vi "General Commands.vi"(8 "error in":errorcluster, 9 "Current Limit":i32=1000, 10 "Action":T1, 11 "VISA in":refnum<visa-resource-name>) -> (0 "error out":errorcluster, 2 "result string":string, 3 "VISA out":refnum<visa-resource-name>)   [LabVIEW 2018]
uses:
  General_lecroy_command.ctl
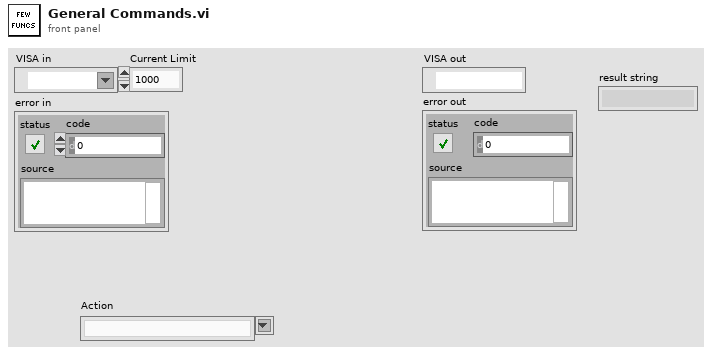
[diagram p1: front panel]
types:
  T1 = typedef "General_lecroy_command.ctl" = string
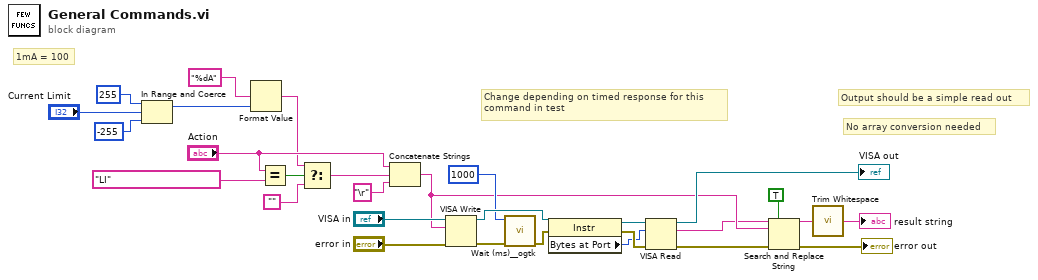
[diagram p0: block diagram]
diagram:
  # "1mA = 100"
  # "Change depending on timed response for this\ncommand in test"
  # "No array conversion needed"
  # "Output should be a simple read out"
  n1 = In Range and Coerce(upper limit=255, x="Current Limit", lower limit=-255 ("upper limit")) -> (coerced(x)=w3:i32)  [unwired: 1 out]
  n2 = Format Value(format string="%dA", value (0)=w3) -> (output string=w7:string)  [unwired: 1 in]
  n3 = Equal?(x="Action", y=T1 "LI") -> (x = y?=w10:bool)
  n4 = Select(t=w7, s=w10, f="") -> (s? t:f=w8:string)
  n5 = Concatenate Strings("Action", w8, "\r") -> (w18:string)
  n6 = VISA Write(VISA resource name="VISA in", write buffer=w18, error in (no error)="error in") -> (VISA resource name out=w24:refnum<visa-resource-name>, error out=w27:errorcluster)  [unwired: 1 out]
  n7 = call <userlib>:"Wait (ms)__ogtk.vi"("error in (no error)"=w27, "milliseconds to wait"=u32 1000) -> ("error out"=w26:errorcluster)  [unwired: 8 in, 1 out]
  n8 = property class="Instr"(reference=w24, error in=w26) -> (reference out=w22:refnum<visa-resource-name>, error out=w25:errorcluster, "Bytes at Port"=w21:u32)
  n9 = VISA Read(VISA resource name=w22, byte count=w21, error in (no error)=w25) -> (VISA resource name out=→"VISA out":refnum<visa-resource-name>, read buffer=w17:string, error out=w15:errorcluster)  [unwired: 1 out]
  n10 = Search and Replace String(replace all?=TRUE ("replace all? (F)"), input string=w17, search string=w18, error in=w15) -> (result string=w13:string, error out=→"error out":errorcluster)  [unwired: 4 in, 2 out]
  n11 = call <vilib>:"Trim Whitespace.vi"("string"=w13) -> ("trimmed string"=→"result string":string)  [unwired: 1 in]
